vi "auto-help-seq-test.vi"() -> ()   [LabVIEW 2019]
uses:
  <vilib>/Rock Robotics/WPI/ThirdParty/JAS_Junk/TrajLib/Enum/DrumSequence_Step_Enum.ctl
  <vilib>/Rock Robotics/WPI/ThirdParty/JAS_Junk/TrajLib/Util_GetTime.vi
  <vilib>/Rock Robotics/WPI/ThirdParty/JAS_Junk/TrajLib/VI/DigSeqLogic_Edge_On.vi
  <vilib>/Rock Robotics/WPI/ThirdParty/JAS_Junk/TrajLib/Timer_New.vi
  <vilib>/Rock Robotics/WPI/ThirdParty/JAS_Junk/TrajLib/DigSeqLogic_SR_FlipFlop.vi
  <vilib>/Rock Robotics/WPI/ThirdParty/JAS_Junk/TrajLib/DigSeqLogic_Off_Delay.vi
  <vilib>/Rock Robotics/WPI/ThirdParty/JAS_Junk/TrajLib/VI/Util_GetTime_U32.vi
  <vilib>/Rock Robotics/WPI/ThirdParty/JAS_Junk/TrajLib/VI/Util_GetTime_U64.vi
  <vilib>/Utility/semaphor.llb/Obtain Semaphore Reference.vi
  <vilib>/Rock Robotics/WPI/ThirdParty/JAS_Junk/TrajLib/Timer_Reset.vi
  <vilib>/Rock Robotics/WPI/ThirdParty/JAS_Junk/TrajLib/VI/Timer_Restart.vi
  <vilib>/Rock Robotics/WPI/ThirdParty/JAS_Junk/TrajLib/Timer_HasPeriodPassedOnce.vi
  <vilib>/Rock Robotics/WPI/ThirdParty/JAS_Junk/TrajLib/Timer_Start.vi
  <vilib>/Rock Robotics/WPI/ThirdParty/JAS_Junk/TrajLib/Timer_Stop.vi
  <vilib>/Rock Robotics/WPI/ThirdParty/JAS_Junk/TrajLib/Trajectory_Library.lvlib
panel:
  out "Output 3":bool
  out "Elapsed Step Time":dbl
  out "New Step":bool
  out "Output 2":bool
  out "Output 1":bool
  out "Error":bool
  out "Seq  Active":bool
  out "Step Number":T1=enum."Initialize"
  in  "milliseconds to wait 2":u32=20
  in  "milliseconds to wait":u32=20
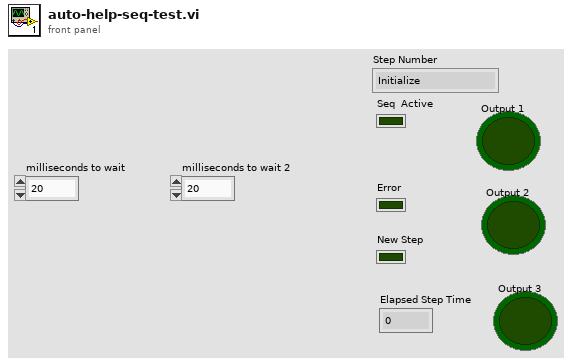
[diagram p1: front panel]
types:
  T1 = typedef "Trajectory_Library.lvlib/DrumSequence_Step_Enum.ctl" = enum16{"Do Nothing", "Step 1", "Step 2", "Step 3", "Step 4", "Step 5", "Step 6", "Step 7", "Step 8", "Step 9", "Step 10", "Step 11", "Step 12", "Step 13", "Step 14", "Step 15", "Step 16", "Step 17", "Step 18", "Step 19", "Step 20", "Step 21", "Step 22", "Step 23", "Step 24", "Step 25", "Step 26", "Step 27", "Step 28", "Step 29", "Step 30", "Step 31", "Step 32", "Cancel", "Initialize", "Error"}
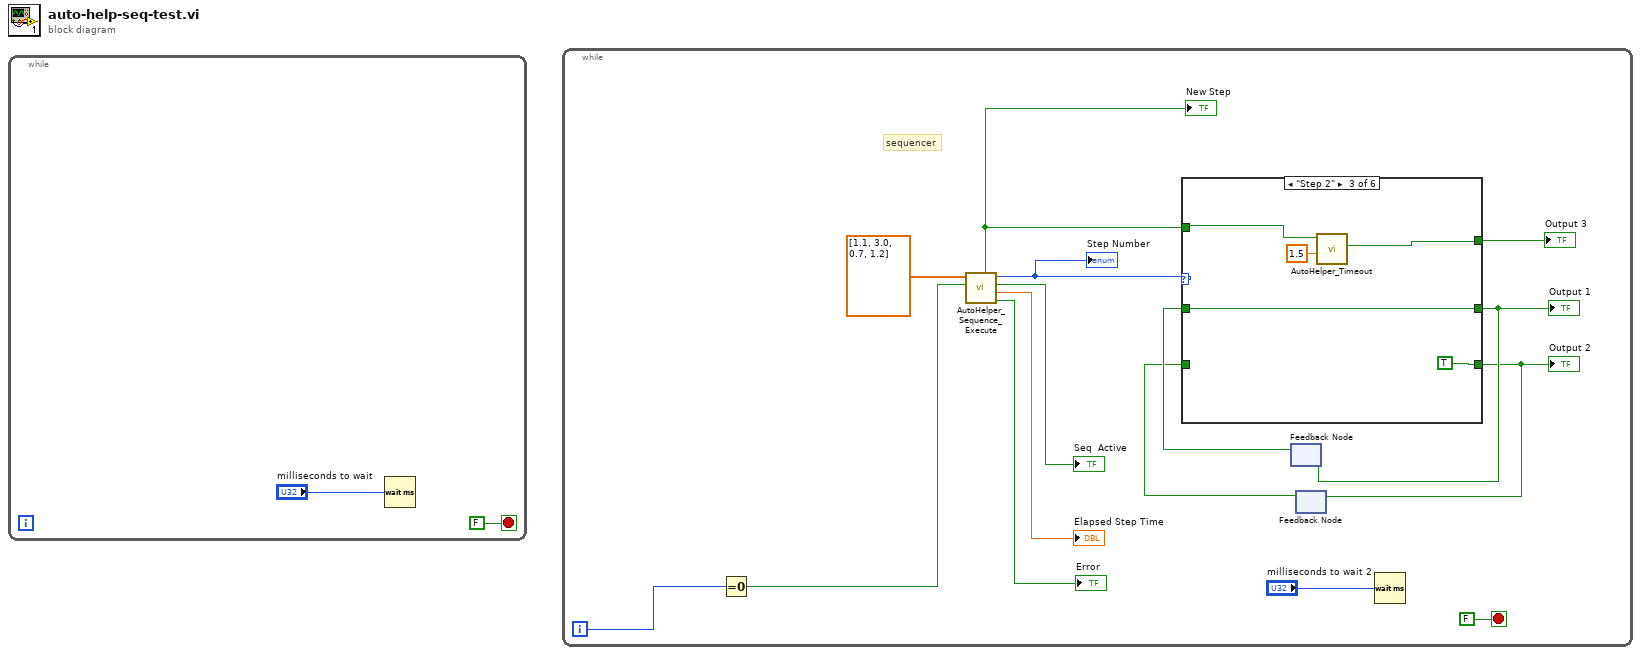
[diagram p0: block diagram]
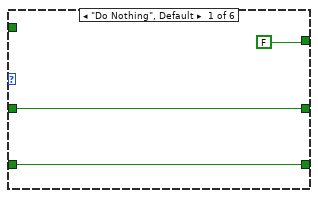
[diagram p2: hidden frame]
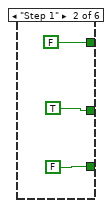
[diagram p3: hidden frame]
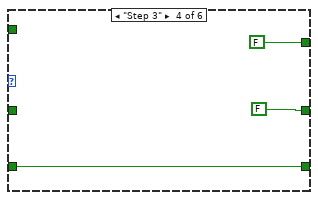
[diagram p4: hidden frame]
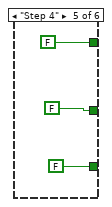
[diagram p5: hidden frame]
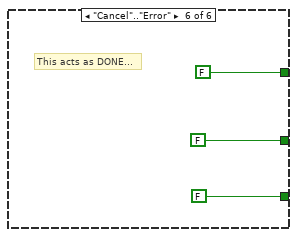
[diagram p6: hidden frame]
diagram:
  n1 = while {
    stop <- FALSE stop-if-true
    n2 = Wait (ms)(milliseconds to wait="milliseconds to wait") -> ()  [unwired: 1 out]
  }
  n3 = while {
    i -> [w11]
    stop <- FALSE stop-if-true
    # "sequencer"
    n4 = Equal To 0?(x=w11) -> (x = 0?=w9:bool)
    n5 = call <vilib>:"AutoHelper_Sequence_Execute.vi"("Initiate"=w9, "Step Times Sec"=dbl[] [1.1, 3.0, 0.7, 1.2]) -> ("Error"=→"Error":bool, "Elapsed Step Time"=→"Elapsed Step Time":dbl, "Seq  Active"=→"Seq  Active":bool, "Step Number State"=w5:T1, "New Step"=w4:bool)  [unwired: 5 in]
    "Step Number" <- w5
    "New Step" <- w4
    n6 = feedback #1() -> (w13:bool)  [unwired: 1 in]
    n7 = feedback #2() -> (w12:bool)  [unwired: 1 in]
    n8 = case shown="\"Step 2\"" w5 {
      tunnel: [w20 TRUE w27 FALSE FALSE FALSE] -> w15
      tunnel: [w19 FALSE TRUE w30 FALSE FALSE] -> w14
      tunnel: w13 -> [w20 _ w27 _ _ _]
      tunnel: w12 -> [w19 _ _ w30 _ _]
      tunnel: w4 -> [_ _ w26 _ _ _]
      tunnel: [FALSE FALSE w24 FALSE FALSE FALSE] -> w3
      frame "Do Nothing", Default {
      }
      frame "Step 1" {
      }
      frame "Step 2" {
        n9 = call <vilib>:"AutoHelper_Timeout.vi"("Timeout Sec"=1.5, "New Step"=w26) -> ("Timeout ALT"=w24:bool)  [unwired: 6 in, 3 out]
      }
      frame "Step 3" {
      }
      frame "Step 4" {
      }
      frame "Cancel".."Error" {
        # "This acts as DONE..."
      }
    }
    "Output 1" <- w15
    "Output 2" <- w14
    "Output 3" <- w3
    n10 = feedback-in #1(w15) -> ()
    n11 = feedback-in #2(w14) -> ()
    n12 = Wait (ms)(milliseconds to wait="milliseconds to wait 2") -> ()  [unwired: 1 out]
  }
